vi "Example Global.vi"() -> ()   [LabVIEW 2015, in "CRDS.lvclass"]
uses:
  Main/CRDS.lvclass
panel:
  in  "Housekeeping":cluster{"Pressure":dbl, "Temperature":dbl}
  in  "RD_Data":dbl[][](array[numeric])
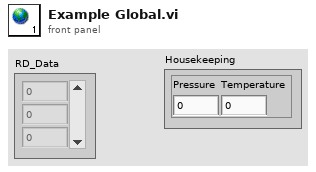
[diagram p1: front panel]
diagram:
